vi "Exercise_2(Main).vi"() -> ()   [LabVIEW 2015]
uses:
  State Defining Enum.ctl
  Enum Defining myDAQ Actions.ctl
panel:
  in  "Stop Button":bool
  out "Number of bits":i32
  out "Number of 1's":i32
  out "output":bool
  out "input":bool
  # "Parity Detector"
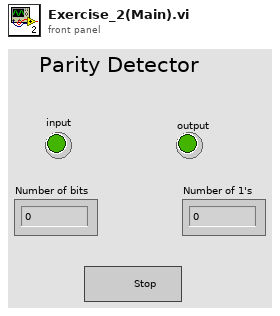
[diagram p1: front panel]
types:
  T1 = typedef "Enum Defining myDAQ Actions.ctl" = enum16{"Initilialize", "Read Reset Button", "Read T, B, P, and C", "Write Output", "Release"}
  T2 = typedef "State Defining Enum.ctl" = enum16{"S0", "S1"}
  T3 = typedef "Enume Defining myDAQ Actions.ctl" = enum16{"Initilialize", "Read Reset Button", "Read Bit Stream", "Write Output", "Release"}
  T4 = typedef "Enum Defining FSM State.ctl" = enum16{"S0", "S1", "S2", "S3"}
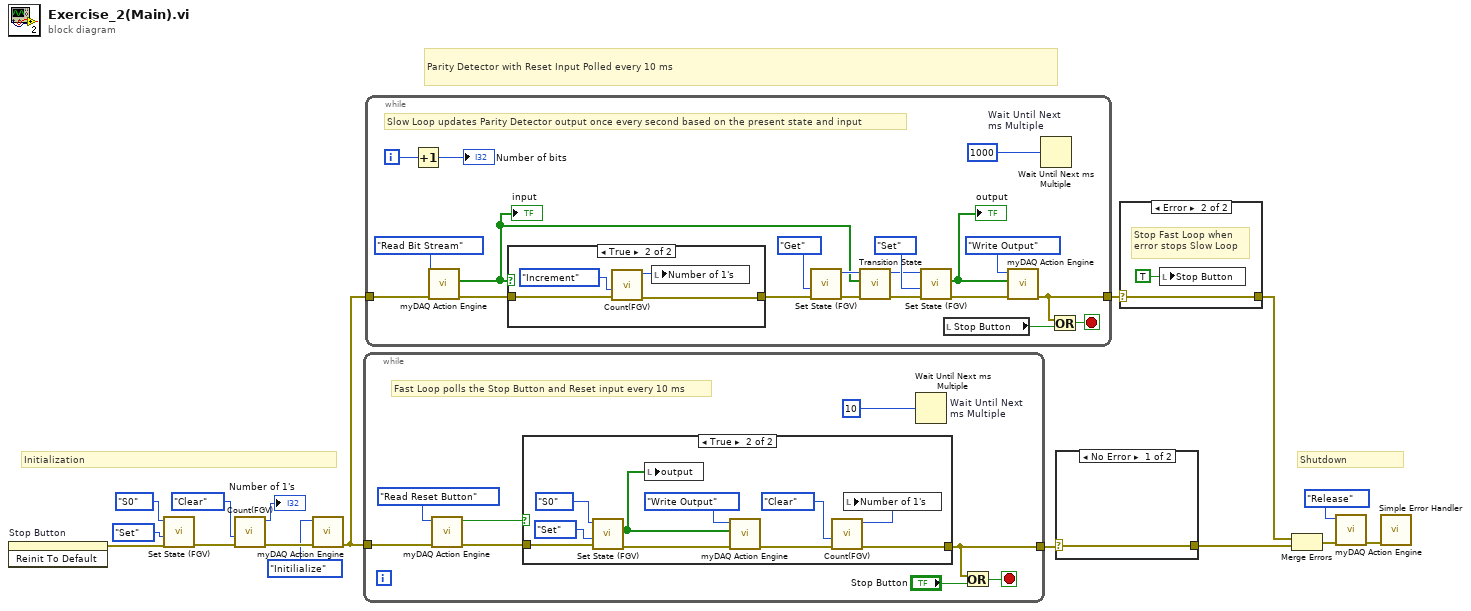
[diagram p0: block diagram]
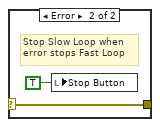
[diagram p2: hidden frame]
diagram:
  # "Shutdown"
  # "Initialization"
  # "Parity Detector with Reset Input Polled every 10 ms"
  n1 = invoke on="Stop Button" class="Bool (strict)" method="Reinit To Default"() -> (error out=w7:errorcluster)  [unwired: 3 in, 2 out]
  n2 = call "Set State (FGV).vi"("Error In"=w7, "Action"=enum16{"Set", "Get"}."Set", "State Input"=State_Defining_Enum."S0" ("Input State")) -> ("Error Out"=w14:errorcluster)  [unwired: 6 in, 2 out]
  n3 = call "Count(FGV).vi"("Error In"=w14, "Action"=enum16{"Clear", "Increment"}."Clear") -> ("Error Out"=w12:errorcluster, "Count"=→"Number of 1's":i32)  [unwired: 8 in]
  n4 = call "myDAQ Action Engine.vi"("Error In"=w12, "Enum Defining myDAQ Action"=Enum_Defining_myDAQ_Actions."Initilialize" ("Enum Defining DIO Action")) -> ("Error Out"=w10:errorcluster)  [unwired: 7 in, 2 out]
  n5 = while {
    tunnel: w10 -> [w23]
    tunnel: [w19] -> w1
    stop <- w21 stop-if-true
    # "Fast Loop polls the Stop Button and Reset input every 10 ms"
    n6 = call "myDAQ Action Engine.vi"("Error In"=w23, "Enum Defining myDAQ Action"=Enum_Defining_myDAQ_Actions."Read Reset Button" ("Enum Defining DIO Action")) -> ("Error Out"=w22:errorcluster, "Reset Button"=w17:bool)  [unwired: 7 in, 1 out]
    n7 = case shown="True" w17 {
      tunnel: w22 -> [w25 w35]
      tunnel: [w25 w29] -> w19
      frame False {
      }
      frame True {
        n8 = call "Set State (FGV).vi"("Error In"=w35, "Action"=enum16{"Set", "Get"}."Set", "State Input"=State_Defining_Enum."S0" ("Input State")) -> ("Error Out"=w32:errorcluster, "Outputs"=w26:bool[])  [unwired: 6 in, 1 out]
        n9 = local write "output"(w26) -> ()
        n10 = call "myDAQ Action Engine.vi"("Error In"=w32, "Outputs U, D"=w26, "Enum Defining myDAQ Action"=Enum_Defining_myDAQ_Actions."Write Output" ("Enum Defining DIO Action")) -> ("Error Out"=w31:errorcluster)  [unwired: 6 in, 2 out]
        n11 = call "Count(FGV).vi"("Error In"=w31, "Action"=enum16{"Clear", "Increment"}."Clear") -> ("Error Out"=w29:errorcluster, "Count"=w28:i32)  [unwired: 8 in]
        n12 = local write "Number of 1's"(w28) -> ()
      }
    }
    n13 = Wait Until Next ms Multiple "Wait Until Next \nms Multiple"(millisecond multiple=u32 10 ("millisecond\nmultiple")) -> ()  [unwired: 1 out]
    n14 = Or(x=w19, y="Stop Button") -> (x .or. y?=w21:bool)
  }
  n15 = while {
    tunnel: w10 -> [w55]
    tunnel: [w40] -> w6
    i -> [w41]
    stop <- w51 stop-if-true
    # "Slow Loop updates Parity Detector output once every second based on the present state and input"
    n16 = Increment(x=w41) -> (x+1=→"Number of bits":i32)
    n17 = call "myDAQ Action Engine.vi"("Error In"=w55, "Enum Defining myDAQ Action"=Enume_Defining_myDAQ_Actions."Read Bit Stream" ("Enum Defining DIO Action")) -> ("Error Out"=w46:errorcluster, "Inputs T, B, nP, C"=w36:bool[])  [unwired: 7 in, 1 out]
    "input" <- w36
    n18 = case shown="True" w36 {
      tunnel: w46 -> [w56 w60]
      tunnel: [w56 w59] -> w45
      frame False {
      }
      frame True {
        n19 = call "Count(FGV).vi"("Error In"=w60, "Action"=enum16{"Clear", "Increment"}."Increment") -> ("Error Out"=w59:errorcluster, "Count"=w57:i32)  [unwired: 8 in]
        n20 = local write "Number of 1's"(w57) -> ()
      }
    }
    n21 = call "Set State (FGV).vi"("Error In"=w45, "Action"=enum16{"Set", "Get"}."Get") -> ("Error Out"=w53:errorcluster, "State Output"=w52:T4)  [unwired: 7 in, 1 out]
    n22 = call "Transition State.vi"("Error In"=w53, "Inputs T,  B, P, C"=w36, "Present  State"=w52) -> ("Error Out"=w48:errorcluster, "Next State"=w49:T4)  [unwired: 7 in]
    n23 = call "Set State (FGV).vi"("Error In"=w48, "Action"=enum16{"Set", "Get"}."Set", "State Input"=w49) -> ("Error Out"=w47:errorcluster, "Outputs"=w37:bool[])  [unwired: 6 in, 1 out]
    "output" <- w37
    n24 = local read "Stop Button"() -> (w43:bool)
    n25 = call "myDAQ Action Engine.vi"("Error In"=w47, "Outputs U, D"=w37, "Enum Defining myDAQ Action"=Enum_Defining_myDAQ_Actions."Write Output" ("Enum Defining DIO Action")) -> ("Error Out"=w40:errorcluster)  [unwired: 6 in, 2 out]
    n26 = Wait Until Next ms Multiple "Wait Until Next \nms Multiple"(millisecond multiple=u32 1000 ("millisecond\nmultiple")) -> ()  [unwired: 1 out]
    n27 = Or(x=w40, y=w43) -> (x .or. y?=w51:bool)
  }
  n28 = case shown="No Error" w1 {
    selector: w1 -> [w61 w63]
    tunnel: [w61 w63] -> w5
    frame No Error {
    }
    frame Error {
      # "Stop Slow Loop when\nerror stops Fast Loop"
      n29 = local write "Stop Button"(TRUE ("Stop Button")) -> ()
    }
  }
  n30 = case shown="Error" w6 {
    selector: w6 -> [w64 w65]
    tunnel: [w64 w65] -> w4
    frame No Error {
    }
    frame Error {
      # "Stop Fast Loop when\nerror stops Slow Loop"
      n31 = local write "Stop Button"(TRUE ("Stop Button")) -> ()
    }
  }
  n32 = Merge Errors(w4, w5) -> (w9:errorcluster)
  n33 = call "myDAQ Action Engine.vi"("Error In"=w9, "Enum Defining myDAQ Action"=Enum_Defining_myDAQ_Actions."Release" ("Enum Defining DIO Action")) -> ("Error Out"=w11:errorcluster)  [unwired: 7 in, 2 out]
  n34 = call <vilib>:"Simple Error Handler.vi"("error in (no error)"=w11) -> ()  [unwired: 4 in, 5 out]
